vi "CreateNewProj.vi"   [LabVIEW 2024]
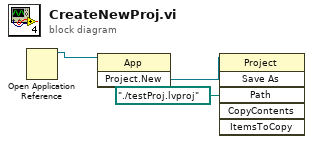
[diagram p0: block diagram]
diagram:
  n1 = Open Application Reference() -> (3:w3:refnum<vi>)  [unwired: 4 in, 1 out]
  n2 = invoke class="App" method="Project.New"(reference=w3) -> ("Project:New"=w2:refnum<vi>)  [unwired: 2 in, 2 out]
  n3 = invoke class="Project" method="Save As"(reference=w2, "Path"=path "./testProj.lvproj") -> ()  [unwired: 4 in, 6 out]
